vi "VI Tree.vi"   [LabVIEW 2014, in "Eurotherm 35xx Series.lvlib"]
doc: "This is the instrument driver for the ET3500 <Eurotherm 3500 series>. The VI Tree displays all the user-callable VIs of the instrument driver in an organized table.\n\nImportant:\nPlease, read controller operation handbook carefully before start using driver. If you have problem with some VI function, check this function with Eurotherm iTools software to be sure, that it is supported by your controller. This fact depends on various configurations of controller, additional modules or types of controller. There is no controller with support of all functions.\n\nNote:\nThis driver doesn't supported settings for all specific parameters of ET3500 instrument series."
uses:
  <instrlib>/Eurotherm 35xx Series/Eurotherm 35xx Series.lvlib
panel:
  # "(c) 2005-2010 NATIONAL INSTRUMENTS.  ALL RIGHTS RESERVED."
  # "SEE DIAGRAM\nFOR VI TREE."
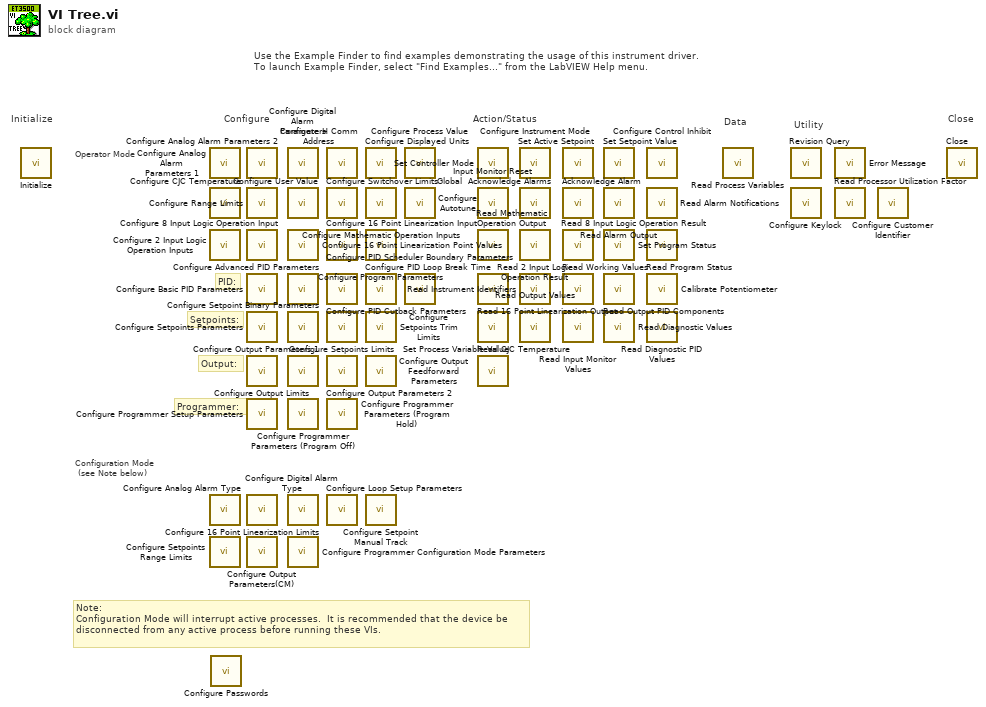
[diagram p0: block diagram]
diagram:
  # "Programmer:"
  # "Output:"
  # "Setpoints:"
  # "PID:"
  # "Configuration Mode\n (see Note below)"
  # "Operator Mode"
  # "Note:\nConfiguration Mode will interrupt active processes.  It is recommended that the device be disconnected from any active process before running these VIs."
  # "Use the Example Finder to find examples demonstrating the usage of this instrument driver.\nTo launch Example Finder, select \"Find Examples...\" from the LabVIEW Help menu."
  # "Configure"
  # "Utility"
  # "Data"
  # "Action/Status"
  # "Close"
  # "Initialize"
  n1 = call <instrlib>:"Initialize.vi"() -> ()  [unwired: 14 in, 2 out]
  n2 = call <instrlib>:"Configure Analog Alarm Parameters 1.vi"() -> ()  [unwired: 14 in, 2 out]
  n3 = call <instrlib>:"Configure CJC Temperature.vi"() -> ()  [unwired: 10 in, 2 out]
  n4 = call <instrlib>:"Configure 2 Input Logic Operation Inputs.vi"() -> ()  [unwired: 10 in, 2 out]
  n5 = call <instrlib>:"Configure Analog Alarm Type.vi"() -> ()  [unwired: 10 in, 2 out]
  n6 = call <instrlib>:"Configure Setpoints Range Limits.vi"() -> ()  [unwired: 10 in, 2 out]
  n7 = call <instrlib>:"Configure Passwords.vi"() -> ()  [unwired: 10 in, 2 out]
  n8 = call <instrlib>:"Configure Analog Alarm Parameters 2.vi"() -> ()  [unwired: 14 in, 2 out]
  n9 = call <instrlib>:"Configure Range Limits.vi"() -> ()  [unwired: 10 in, 2 out]
  n10 = call <instrlib>:"Configure 8 Input Logic Operation Input.vi"() -> ()  [unwired: 10 in, 2 out]
  n11 = call <instrlib>:"Configure Basic PID Parameters.vi"() -> ()  [unwired: 14 in, 2 out]
  n12 = call <instrlib>:"Configure Setpoints Parameters.vi"() -> ()  [unwired: 10 in, 2 out]
  n13 = call <instrlib>:"Configure Output Limits.vi"() -> ()  [unwired: 10 in, 2 out]
  n14 = call <instrlib>:"Configure Programmer Setup Parameters.vi"() -> ()  [unwired: 14 in, 2 out]
  n15 = call <instrlib>:"Configure Digital Alarm Type.vi"() -> ()  [unwired: 10 in, 2 out]
  n16 = call <instrlib>:"Configure Output Parameters(CM).vi"() -> ()  [unwired: 10 in, 2 out]
  n17 = call <instrlib>:"Configure Digital Alarm Parameters.vi"() -> ()  [unwired: 14 in, 2 out]
  n18 = call <instrlib>:"Configure User Value.vi"() -> ()  [unwired: 10 in, 2 out]
  n19 = call <instrlib>:"Configure 16 Point Linearization Point Values.vi"() -> ()  [unwired: 10 in, 2 out]
  n20 = call <instrlib>:"Configure Advanced PID Parameters.vi"() -> ()  [unwired: 10 in, 2 out]
  n21 = call <instrlib>:"Configure Setpoint Binary Parameters.vi"() -> ()  [unwired: 10 in, 2 out]
  n22 = call <instrlib>:"Configure Output Parameters 1.vi"() -> ()  [unwired: 14 in, 2 out]
  n23 = call <instrlib>:"Configure Programmer Parameters (Program Off).vi"() -> ()  [unwired: 10 in, 2 out]
  n24 = call <instrlib>:"Configure 16 Point Linearization Limits.vi"() -> ()  [unwired: 14 in, 2 out]
  n25 = call <instrlib>:"Configure Programmer Configuration Mode Parameters.vi"() -> ()  [unwired: 14 in, 2 out]
  n26 = call <instrlib>:"Configure H Comm Address.vi"() -> ()  [unwired: 10 in, 2 out]
  n27 = call <instrlib>:"Configure Switchover Limits.vi"() -> ()  [unwired: 10 in, 2 out]
  n28 = call <instrlib>:"Configure 16 Point Linearization Input.vi"() -> ()  [unwired: 10 in, 2 out]
  n29 = call <instrlib>:"Configure PID Cutback Parameters.vi"() -> ()  [unwired: 10 in, 2 out]
  n30 = call <instrlib>:"Configure Setpoints Limits.vi"() -> ()  [unwired: 10 in, 2 out]
  n31 = call <instrlib>:"Configure Output Parameters 2.vi"() -> ()  [unwired: 14 in, 2 out]
  n32 = call <instrlib>:"Configure Programmer Parameters (Program Hold).vi"() -> ()  [unwired: 14 in, 2 out]
  n33 = call <instrlib>:"Configure Loop Setup Parameters.vi"() -> ()  [unwired: 14 in, 2 out]
  n34 = call <instrlib>:"Configure Displayed Units.vi"() -> ()  [unwired: 10 in, 2 out]
  n35 = call <instrlib>:"Configure Mathematic Operation Inputs.vi"() -> ()  [unwired: 10 in, 2 out]
  n36 = call <instrlib>:"Configure Program Parameters.vi"() -> ()  [unwired: 10 in, 2 out]
  n37 = call <instrlib>:"Configure PID Loop Break Time.vi"() -> ()  [unwired: 10 in, 2 out]
  n38 = call <instrlib>:"Configure Setpoints Trim Limits.vi"() -> ()  [unwired: 10 in, 2 out]
  n39 = call <instrlib>:"Configure Output Feedforward Parameters.vi"() -> ()  [unwired: 10 in, 2 out]
  n40 = call <instrlib>:"Configure Setpoint Manual Track.vi"() -> ()  [unwired: 10 in, 2 out]
  n41 = call <instrlib>:"Configure Process Value.vi"() -> ()  [unwired: 10 in, 2 out]
  n42 = call <instrlib>:"Configure Autotune.vi"() -> ()  [unwired: 10 in, 2 out]
  n43 = call <instrlib>:"Configure PID Scheduler Boundary Parameters.vi"() -> ()  [unwired: 10 in, 2 out]
  n44 = call <instrlib>:"Set Controller Mode.vi"() -> ()  [unwired: 10 in, 2 out]
  n45 = call <instrlib>:"Input Monitor Reset.vi"() -> ()  [unwired: 10 in, 2 out]
  n46 = call <instrlib>:"Read Mathematic Operation Output.vi"() -> ()  [unwired: 9 in, 3 out]
  n47 = call <instrlib>:"Read 16 Point Linearization Output.vi"() -> ()  [unwired: 9 in, 3 out]
  n48 = call <instrlib>:"Set Process Variable Value.vi"() -> ()  [unwired: 10 in, 2 out]
  n49 = call <instrlib>:"Read CJC Temperature.vi"() -> ()  [unwired: 9 in, 3 out]
  n50 = call <instrlib>:"Configure Instrument Mode.vi"() -> ()  [unwired: 10 in, 2 out]
  n51 = call <instrlib>:"Global  Acknowledge Alarms.vi"() -> ()  [unwired: 10 in, 2 out]
  n52 = call <instrlib>:"Read 2 Input Logic Operation Result.vi"() -> ()  [unwired: 9 in, 3 out]
  n53 = call <instrlib>:"Read Instrument Identifiers.vi"() -> ()  [unwired: 6 in, 6 out]
  n54 = call <instrlib>:"Read Output Values.vi"() -> ()  [unwired: 7 in, 5 out]
  n55 = call <instrlib>:"Set Active Setpoint.vi"() -> ()  [unwired: 10 in, 2 out]
  n56 = call <instrlib>:"Acknowledge Alarm.vi"() -> ()  [unwired: 10 in, 2 out]
  n57 = call <instrlib>:"Read 8 Input Logic Operation Result.vi"() -> ()  [unwired: 9 in, 3 out]
  n58 = call <instrlib>:"Read Working Values.vi"() -> ()  [unwired: 8 in, 4 out]
  n59 = call <instrlib>:"Read Input Monitor Values.vi"() -> ()  [unwired: 7 in, 5 out]
  n60 = call <instrlib>:"Set Setpoint Value.vi"() -> ()  [unwired: 10 in, 2 out]
  n61 = call <instrlib>:"Read Alarm Output.vi"() -> ()  [unwired: 9 in, 3 out]
  n62 = call <instrlib>:"Set Program Status.vi"() -> ()  [unwired: 10 in, 2 out]
  n63 = call <instrlib>:"Read Output PID Components.vi"() -> ()  [unwired: 7 in, 5 out]
  n64 = call <instrlib>:"Read Diagnostic Values.vi"() -> ()  [unwired: 7 in, 5 out]
  n65 = call <instrlib>:"Configure Control Inhibit.vi"() -> ()  [unwired: 10 in, 2 out]
  n66 = call <instrlib>:"Read Alarm Notifications.vi"() -> ()  [unwired: 8 in, 4 out]
  n67 = call <instrlib>:"Read Program Status.vi"() -> ()  [unwired: 8 in, 4 out]
  n68 = call <instrlib>:"Calibrate Potentiometer.vi"() -> ()  [unwired: 10 in, 2 out]
  n69 = call <instrlib>:"Read Diagnostic PID Values.vi"() -> ()  [unwired: 7 in, 5 out]
  n70 = call <instrlib>:"Read Process Variables.vi"() -> ()  [unwired: 8 in, 4 out]
  n71 = call <instrlib>:"Revision Query.vi"() -> ()  [unwired: 12 in, 4 out]
  n72 = call <instrlib>:"Configure Keylock.vi"() -> ()  [unwired: 10 in, 2 out]
  n73 = call <instrlib>:"Error Message.vi"() -> ()  [unwired: 11 in, 5 out]
  n74 = call <instrlib>:"Read Processor Utilization Factor.vi"() -> ()  [unwired: 9 in, 3 out]
  n75 = call <instrlib>:"Configure Customer Identifier.vi"() -> ()  [unwired: 10 in, 2 out]
  n76 = call <instrlib>:"Close.vi"() -> ()  [unwired: 15 in, 1 out]
